vi "Reset ROI.vi"(8 "error in (no error)":errorcluster, 11 "TG Base Graph in":refnum<class "TG Base Graph.lvclass">) -> (0 "error out":errorcluster, 3 "TG Base Graph out":refnum<class "TG Base Graph.lvclass">)   [LabVIEW 2023, in "TG Base Graph.lvclass"]
uses:
  TG Base Graph.lvclass
  TG Base Graph.lvclass/TG Base Graph.ctl
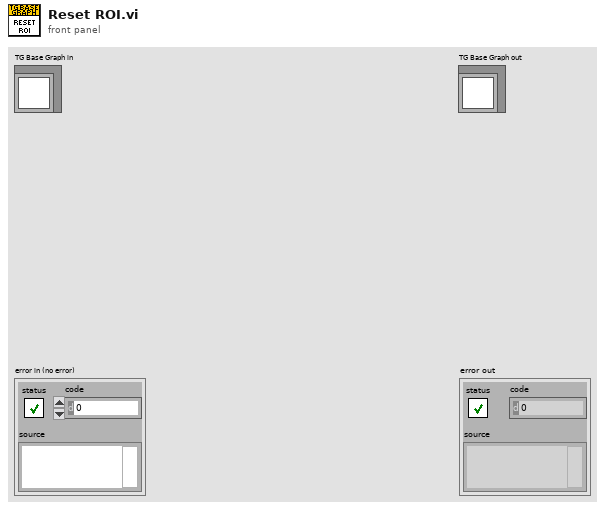
[diagram p1: front panel]
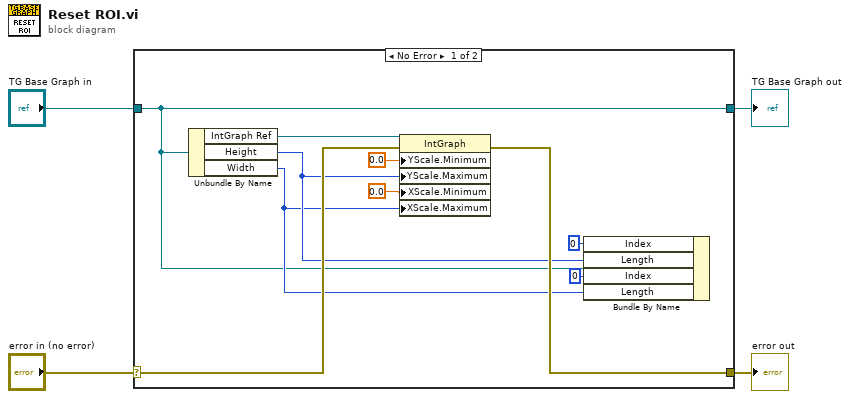
[diagram p0: block diagram]
diagram:
  n1 = case shown="No Error" "error in (no error)" {
    selector: "error in (no error)" -> [w13 w16]
    tunnel: [w10 w16] -> w3
    tunnel: [w5 w15] -> w1
    tunnel: "TG Base Graph in" -> [w5 w15]
    frame No Error {
      n2 = Unbundle By Name(w5) -> ("IntGraph Ref"=w14:refnum<vi>, "Height"=w7:u32, "Width"=w6:u32)
      n3 = property class="IntGraph"(reference=w14, error in=w13, "YScale.Minimum"=0.0 ("Y Scale.Range:Minimum"), "YScale.Maximum"=w7, "XScale.Minimum"=0.0 ("X Scale.Range:Minimum"), "XScale.Maximum"=w6) -> (error out=w10:errorcluster)  [unwired: 1 out]
      n4 = Bundle By Name(cluster=w5, "Index"=u32 0 ("ROI XY.ROI X.Index"), "Length"=w7, "Index"=u32 0 ("ROI XY.ROI Y.Index"), "Length"=w6) -> ()  [unwired: 1 out]
    }
    frame Error {
    }
  }
  "error out" <- w3
  "TG Base Graph out" <- w1
